vi "Populate Subpanels.vi"(8 "error in (no error)":errorcluster, 9 "View Labels (optional)":string[](array[string]), 10 "Views":refnum<class "Message Enqueuer.lvclass">[](array[class]), 11 "QuadViewManager In":refnum<class "QuadViewManager.lvclass">) -> (0 "error out":errorcluster, 3 "QuadViewManager Out":refnum<class "QuadViewManager.lvclass">)   [LabVIEW 2015, in "QuadViewManager.lvlib" / "QuadViewManager.lvclass"]
doc: "<License>\nCopyright © 2017 Composed Systems, LLC | All rights reserved\nwww.composed.io\n\nAuthor: Ethan Stern <ethan.stern@composed.io>\n\nThis software is provided \"AS IS\" WITHOUT WARRANTIES, either express or implied, AND IS FOR EDUCATIONAL PURPOSES ONLY.\n</License>"
uses:
  QuadViewManager.lvclass
  <vilib>/ActorFramework/Message Enqueuer/Message Enqueuer.lvclass
  QuadViewManager.lvclass/QuadViewManager.ctl
  Framework/IViewable/IViewable Messages/Insert View Msg/Insert View Msg.lvclass/Insert View Msg.ctl
  <vilib>/ActorFramework/Message Enqueuer/Message Enqueuer.lvclass/Message Enqueuer.ctl
  <vilib>/ActorFramework/Message Enqueuer/Enqueue.vi
  <vilib>/ActorFramework/Message Priority Queue/Priority Enqueue.vi
  Framework/IViewManager/IViewManager/IViewManager.lvclass
  Framework/IViewable/IViewable Messages/Insert View Msg/Insert View Msg.lvclass
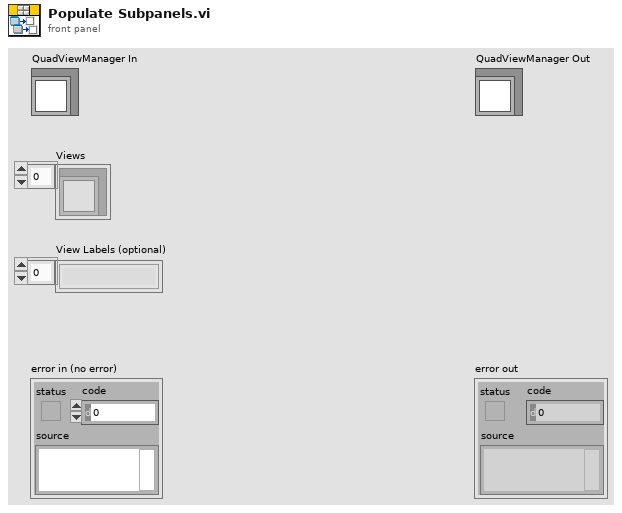
[diagram p1: front panel]
types:
  T1 = typedef "ProtectedSubpanel.lvlibp/ProtectedSubpanel.lvclass/Protected Subpanel Reference.ctl" = refnum<data-value>
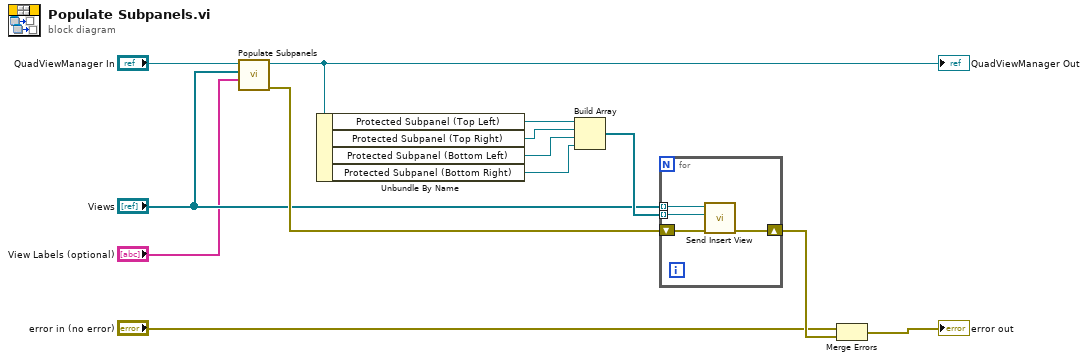
[diagram p0: block diagram]
diagram:
  n1 = call-parent "Populate Subpanels.vi"("View Labels (optional)"="View Labels (optional)", "Views"="Views", "IViewManager In"="QuadViewManager In") -> ("error out"=w4:errorcluster, "IViewManager Out"=w3:refnum<class "QuadViewManager.lvclass">)  [unwired: 7 in]
  "QuadViewManager Out" <- w3
  n2 = Unbundle By Name(w3) -> ("Protected Subpanel (Top Left)"=w12:T1, "Protected Subpanel (Top Right)"=w9:T1, "Protected Subpanel (Bottom Left)"=w10:T1, "Protected Subpanel (Bottom Right)"=w11:T1)
  n3 = Build Array(w12, w9, w10, w11) -> (w8:T1[])
  n4 = for {
    tunnel: w8 -> [w17] mode=indexing
    shift-right: [w16] -> w7
    shift-left: w4 -> [w15]
    tunnel: "Views" -> [w14] mode=indexing
    n5 = call "Send Insert View.vi"("error in (no error)"=w15, "Protected Subpanel"=w17, "Message Enqueuer"=w14) -> ("error out"=w16:errorcluster)  [unwired: 7 in, 1 out]
  }
  n6 = Merge Errors("error in (no error)", w7) -> (→"error out":errorcluster)
